vi "Write Report Folder.vi"(8 "error in (no error)":errorcluster, 10 "Report Folder":string, 11 "Sequencer Module configuration in":refnum<class "Sequencer Module configuration.lvclass">) -> (0 "error out":errorcluster, 3 "Sequencer Module configuration out":refnum<class "Sequencer Module configuration.lvclass">)   [LabVIEW 2015, in "Sequencer Module configuration.lvclass"]
uses:
  Sequencer Module configuration.lvclass
  Sequencer Module configuration.lvclass/Sequencer Module configuration.ctl
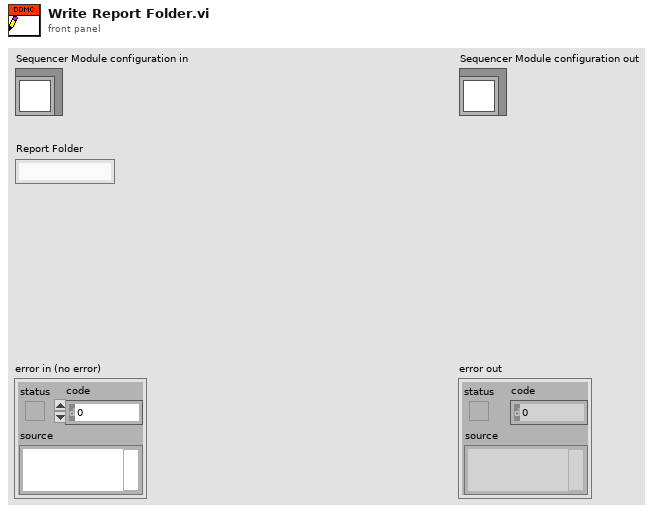
[diagram p1: front panel]
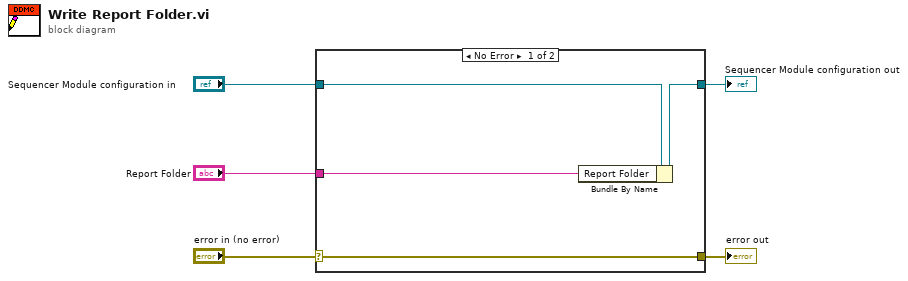
[diagram p0: block diagram]
diagram:
  n1 = case shown="No Error" "error in (no error)" {
    selector: "error in (no error)" -> [w9 w10]
    tunnel: [w9 w10] -> w4
    tunnel: [w7 w11] -> w2
    tunnel: "Sequencer Module configuration in" -> [w8 w11]
    tunnel: "Report Folder" -> [w6 _]
    frame No Error {
      n2 = Bundle By Name(cluster=w8, "Report Folder"=w6) -> (w7:refnum<class "Sequencer Module configuration.lvclass">)
    }
    frame Error {
    }
  }
  "error out" <- w4
  "Sequencer Module configuration out" <- w2
